vi "Array-Rotate and Insert (2D).vi"(0 "Array in":dbl[][](array[numeric]), 7 "Value":dbl[](array[numeric])) -> (4 "Array out":dbl[][](array[numeric]))   [LabVIEW 2020]
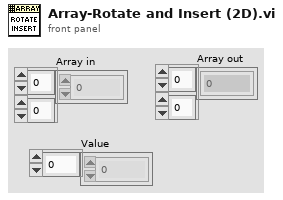
[diagram p1: front panel]
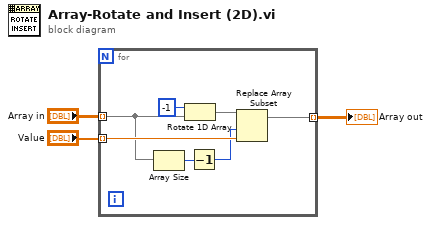
[diagram p0: block diagram]
diagram:
  n1 = for {
    tunnel: "Value" -> [w10] mode=indexing
    tunnel: [w8] -> w2 mode=indexing
    tunnel: "Array in" -> [w4] mode=indexing
    n2 = Array Size(array=w4) -> (size(s)=w5:i32)
    n3 = Rotate 1D Array(1:w4, 2:-1 ("n")) -> (0:w7:dbl[])
    n4 = Decrement(x=w5) -> (x-1=w9:i32)
    n5 = Replace Array Subset(array=w7, new element=w10, index=w9) -> (w8:dbl[])
  }
  "Array out" <- w2
